vi "PWM5.vi"() -> ()   [LabVIEW 2019]
uses:
  <vilib>/rvi/Emulation/niFpgaGetClockAttributes.vi
  <vilib>/rvi/Emulation/niFpgaSctlEmulationGetInTimedLoop.vi
  <vilib>/rvi/Emulation/niFpgaEmulationReportErrorSimple.vi
  <vilib>/rvi/eio/common/nirviEmuTemplateMethod_errors.vi
  <vilib>/rvi/Emulation/niFpgaCriticalErrorInLSC.vi
  <vilib>/eio/EIONode/EIONode.xnode
panel:
  out "x-1":u32
  out "波形图表":u32(graph)
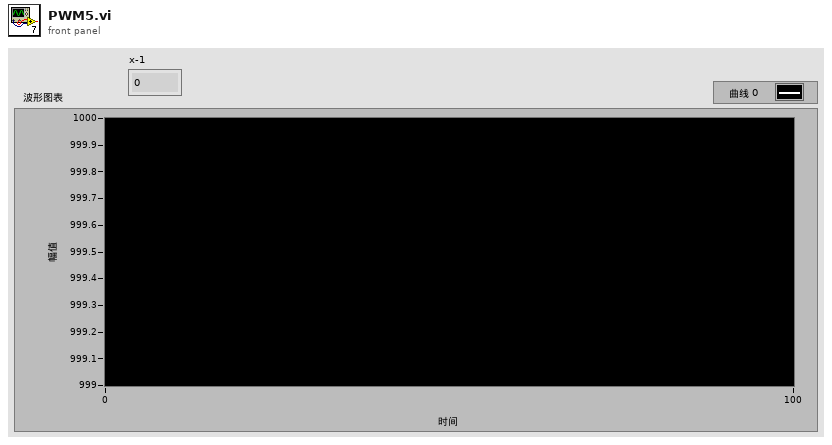
[diagram p1: front panel]
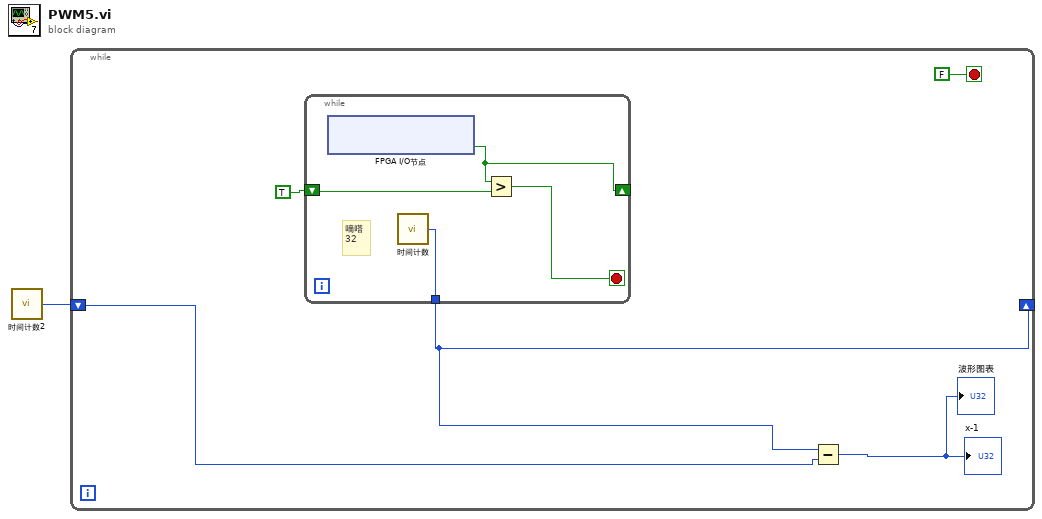
[diagram p0: block diagram]
diagram:
  n1 = call "时间计数2"() -> ("Tick Count(Ticks)"=w1:u32)
  n2 = while {
    shift-right: [w4] -> _
    shift-left: w1 -> [w3]
    stop <- FALSE stop-if-true
    n3 = while {
      shift-right: [w9] -> _
      shift-left: TRUE -> [w10]
      tunnel: [w7] -> w4
      stop <- w8 stop-if-true
      # "嘀嗒\n32"
      n4 = xnode "FPGA I/O节点"() -> ("ConnectorB/DIO0"=w9:bool)  [unwired: 1 in, 1 out]
      n5 = call "时间计数"() -> ("Tick Count(Ticks)"=w7:u32)
      n6 = Greater?(x=w9, y=w10) -> (0:w8:bool)
    }
    n7 = Subtract(x=w4, y=w3) -> (x-y=→"x-1" →"波形图表":u32)
  }
